vi "VNORESET to 2.85V.vi"(8 "error in":errorcluster) -> (0 "error out":errorcluster, 2 "Pass/Fail":bool)   [LabVIEW 2009]
uses:
  <vilib>/Instr/_visa.llb/VISA Configure Serial Port (Instr).vi
  Global/Global 1.vi
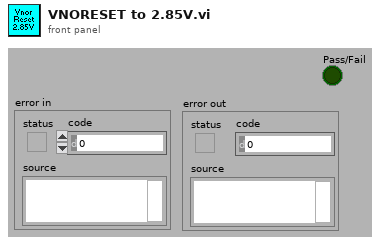
[diagram p1: front panel]
types:
  T1 = enum16{"lock key", "POwer OFF", "Power ON", "SET Volt and Current"}
  T2 = cluster{"VHEATFUSENOLOADMIN":string, "VHEATFUSELOADMAX":string, "VOVERRIDEDIODEMIN":string, "TDIFFMAX":string, "MEASFREQMAX":string, "MEASFREQMIN":string, "VOVER":string, "VMIDDLE":string, "VUNDER":string, "VNORESET":string, "VRESET":string, "WAITPING":string, "LRFID":string, "RFIDUID":string, "EXTEESIZE":string, "LCUTYPE":string, "LCUSUBTYPE":string, "TEVN":string, "BOOTVER":string, "APPVER":string, "ISLEEPMAX":string, "TSLEEP":string, "APPWAIT":string, "DBWAIT":string}
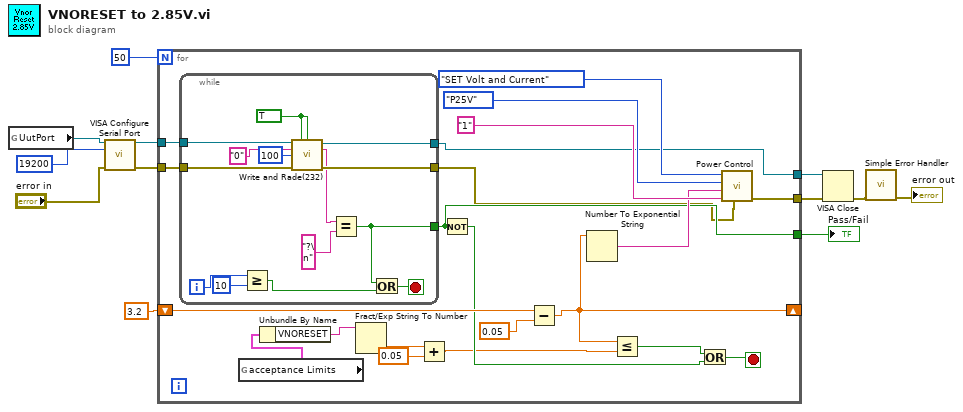
[diagram p0: block diagram]
diagram:
  n1 = global read "Global 1.vi" "UutPort"() -> (w7:refnum<visa-resource-name>)
  n2 = call-poly "VISA Configure Serial Port"("VISA resource name"=w7, "baud rate (9600)"=u32 19200, "error in (no error)"="error in") -> ("VISA resource name out"=w8:refnum<visa-resource-name>, "error out"=w9:errorcluster)  [unwired: 3 in, 8 out]
  n3 = for {
    N: 50 -> [_]
    shift-right: [w19] -> _
    shift-left: 3.2 ("x") -> [w33]
    tunnel: [w23] -> w10
    tunnel: [w24] -> w4
    tunnel: w9 -> [w22]
    tunnel: w8 -> [w21]
    tunnel: [w18] -> w3
    stop <- w27 stop-if-true
    n4 = while {
      tunnel: [w43] -> w23
      tunnel: w22 -> [w40]
      tunnel: w21 -> [w39]
      tunnel: [w37] -> w20
      tunnel: [w36] -> w18
      i -> [w46]
      stop <- w44 stop-if-true
      w38 = TRUE ("write")
      n5 = Greater Or Equal?(x=w46, y=10) -> (x >= y?=w42:bool)
      n6 = call "Write and Rade(232).vi"("VISA resource name in"=w39, "write"=w38, "read"=w38, "string to write"="0", "ms delay"=u32 100, "error in"=w40) -> ("VISA resource name out"=w36:refnum<visa-resource-name>, "read string"=w35:string, "error out"=w37:errorcluster)  [unwired: 2 in, 5 out]
      n7 = Equal?(x=w35, y="?\n") -> (x = y?=w43:bool)
      n8 = Or(x=w43, y=w42) -> (x .or. y?=w44:bool)
    }
    n9 = global read "Global 1.vi" "acceptance Limits"() -> (w17:T2)
    n10 = Unbundle By Name(w17) -> ("VNORESET"=w16:string)
    n11 = Fract/Exp String To Number(string=w16) -> (number=w15:dbl)  [unwired: 4 out]
    n12 = Add(x=w15, y=0.05) -> (x+y=w13:dbl)
    n13 = Not(x=w23) -> (.not. x?=w25:bool)
    n14 = Subtract(x=w33, y=0.05) -> (x-y=w19:dbl)
    n15 = Number To Exponential String(number=w19) -> (E-format string=w28:string)  [unwired: 3 out]
    n16 = Less Or Equal?(x=w19, y=w13) -> (x <= y?=w26:bool)
    n17 = Or(x=w26, y=w25) -> (x .or. y?=w27:bool)
    n18 = call "Power Control.vi"("error in"=w20, "Current"="1", "Voltage"=w28, "Channel"=enum16{"P6V", "P25V", "N25V"}."P25V", "command"=T1."SET Volt and Current") -> ("error out"=w24:errorcluster)  [unwired: 6 out]
  }
  "Pass/Fail" <- w10
  n19 = VISA Close(VISA resource name=w3, error in (no error)=w4) -> (error out=w2:errorcluster)
  n20 = call <vilib>:"Simple Error Handler.vi"("error in (no error)"=w2) -> ("error out"=→"error out":errorcluster)  [unwired: 1 in, 7 out]
